vi "PostInstrument.vi"(8 "error in (no error)":errorcluster, 10 "Instrument":T1, 11 "ByteGSWebAPI-V0 in":refnum<class "ByteGSWebAPI-V0.lvclass">) -> (0 "error out":errorcluster, 3 "ByteGSWebAPI-V0 out":refnum<class "ByteGSWebAPI-V0.lvclass">)   [LabVIEW 2019, in "ByteGSWebAPI-V0.lvclass"]
uses:
  ByteGSWebAPI-V0.lvclass
  1f9a4a84-1e23-43aa-b54f-cc03f7d81dac.vi
  Cntrls/SingleInstrument.ctl
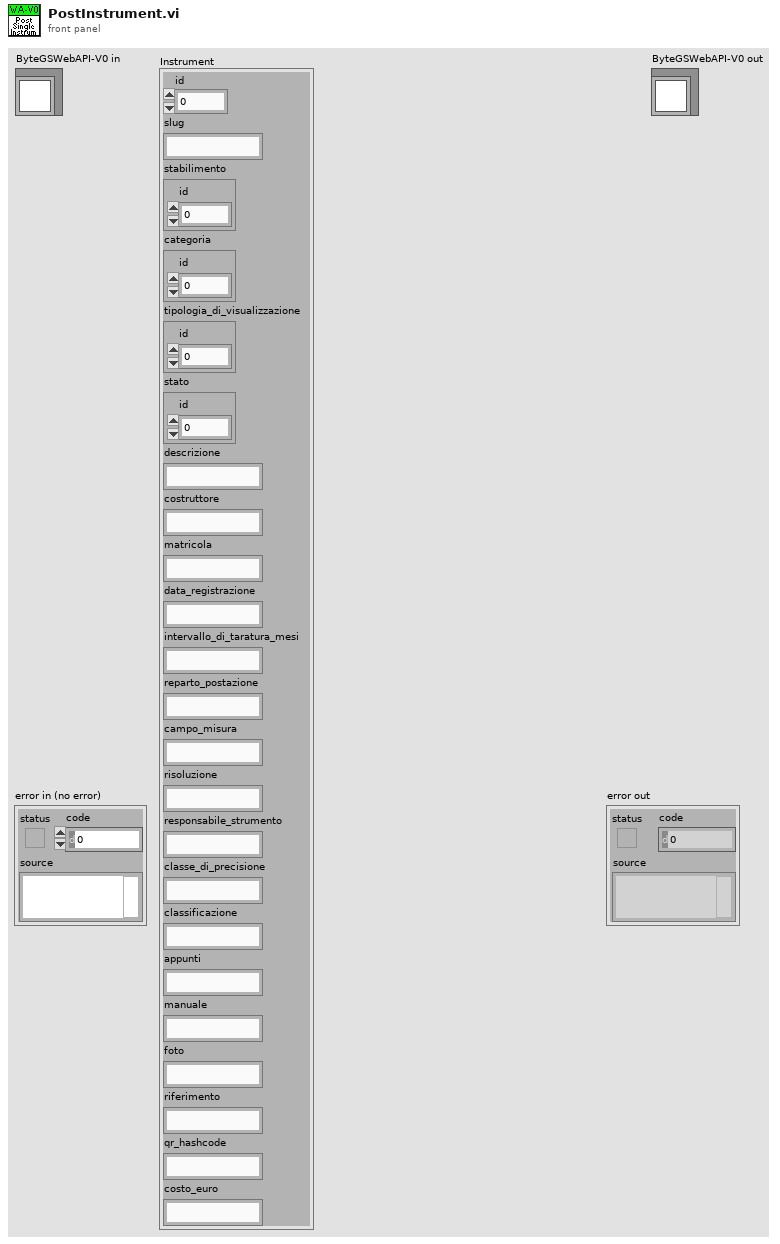
[diagram p1: front panel]
types:
  T1 = typedef "ByteGSWebAPI-V0.lvclass/SingleInstrument.ctl" = cluster{"id":i32, "slug":string, "stabilimento":cluster{"id":dbl}, "categoria":cluster{"id":dbl}, "tipologia_di_visualizzazione":cluster{"id":dbl}, "stato":cluster{"id":dbl}, "descrizione":string, "costruttore":string, "matricola":string, "data_registrazione":string, "intervallo_di_taratura_mesi":string, "reparto_postazione":string, "campo_misura":string, "risoluzione":string, "responsabile_strumento":string, "classe_di_precisione":string, "classificazione":string, "appunti":string, "manuale":string, "foto":string, "riferimento":string, "qr_hashcode":string, "costo_euro":string}
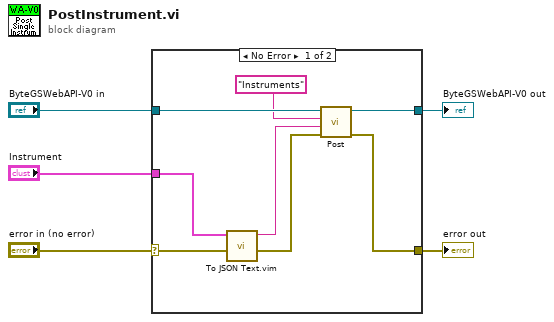
[diagram p0: block diagram]
diagram:
  n1 = case shown="No Error" "error in (no error)" {
    selector: "error in (no error)" -> [w10 w15]
    tunnel: [w6 w15] -> w4
    tunnel: [w13 w14] -> w2
    tunnel: "ByteGSWebAPI-V0 in" -> [w12 w14]
    tunnel: "Instrument" -> [w11 _]
    frame No Error {
      n2 = call "To JSON Text.vim"("error in (no error)"=w10, "Anything"=w11) -> ("error out"=w9:errorcluster, "<JSON>"=w8:string)  [unwired: 8 in]
      n3 = call "Post.vi"("error in (no error)"=w9, "Buffer"=w8, "Request"="Instruments", "ByteGSWebAPI-V0 in"=w12) -> ("error out"=w6:errorcluster, "ByteGSWebAPI-V0 out"=w13:refnum<class "ByteGSWebAPI-V0.lvclass">)  [unwired: 4 in, 2 out]
    }
    frame Error {
    }
  }
  "error out" <- w4
  "ByteGSWebAPI-V0 out" <- w2
